vi "niDTS BT INSTR TX Configure ModAcc.vi"(8 "error in (no error)":errorcluster, 11 "niDTS BT INSTR TX in":refnum<class "niDTS BT INSTR TX.lvclass">) -> (0 "error out":errorcluster, 3 "niDTS BT INSTR TX out":refnum<class "niDTS BT INSTR TX.lvclass">)   [LabVIEW 2015, in "niDTS BT.lvlib" / "niDTS BT INSTR TX.lvclass"]
doc: "Sets:\n\n* TriggerThreshold\n* Trigger Source\n* MinQuietTimeDuration\n* TriggerTimeout"
uses:
  niDTS BT INSTR TX.lvclass
  niDTS BT INSTR TX.lvclass/niDTS BT INSTR TX.ctl
  RiviInstDriver/niRfsaBT/Objects/niRfsaBt.lvclass
  RiviInstDriver/InstDriver/Objects/InstDriver.lvclass
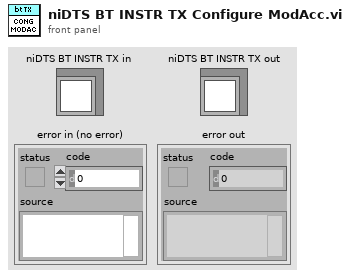
[diagram p1: front panel]
types:
  T1 = typedef "niRfsaBT.lvclass/niRfsaBT INC Handle.ctl" = refnum<data-value>
  T2 = typedef "niDTS BT.lvlib/niDTS BT Tx Test INC Modulation Characteristics.ctl" = enum16{"DF1", "DF2", "BOTH"}
  T3 = enum16{"RMS", "LOG", "SCALAR", "MAX", "MIN", "VECTOR"}
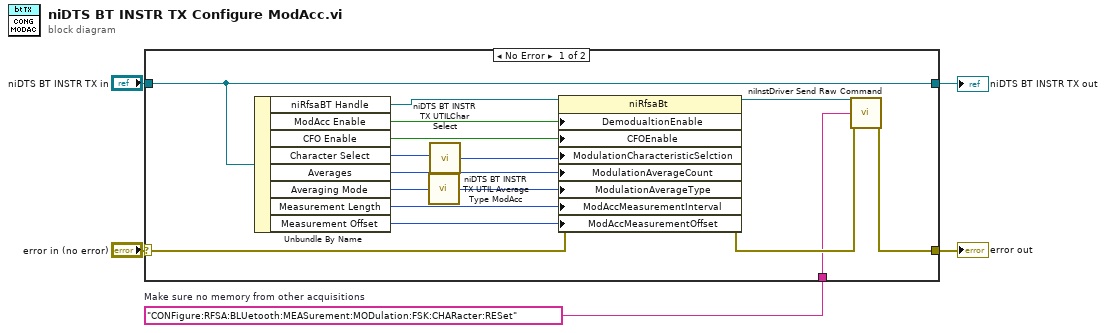
[diagram p0: block diagram]
diagram:
  w1 = "CONFigure:RFSA:BLUetooth:MEASurement:MODulation:FSK:CHARacter:RESet"  # Make sure no memory from other acquisitions
  n1 = case shown="No Error" "error in (no error)" {
    selector: "error in (no error)" -> [w21 w23]
    tunnel: [w7 w23] -> w4
    tunnel: "niDTS BT INSTR TX in" -> [w19 w22]
    tunnel: [w19 w22] -> w2
    tunnel: w1 -> [w6 _]
    frame No Error {
      n2 = Unbundle By Name(w19) -> ("niRfsaBT Handle"=w20:T1, "ModAcc Enable"=w18:bool, "CFO Enable"=w17:bool, "Character Select"=w15:T2, "Averages"=w16:i32, "Averaging Mode"=w14:T3, "Measurement Length"=w13:i32, "Measurement Offset"=w12:i32)
      n3 = call "niDTS BT INSTR TX UTIL Average Type ModAcc.vi"("Average In"=w14) -> ("Average Out"=w10:enum16{"RMS", "MAX", "MIN"})  [unwired: 14 in]
      n4 = call "niDTS BT INSTR TX UTILChar Select.vi"("Character Select"=w15) -> ("ModulationCharacteristicSelction"=w11:enum16{"DF1", "DF2"})  [unwired: 14 in]
      n5 = property class="niRfsaBt"(reference=w20, error in=w21, "DemodualtionEnable"=w18, "CFOEnable"=w17, "ModulationCharacteristicSelction"=w11, "ModulationAverageCount"=w16, "ModulationAverageType"=w10, "ModAccMeasurementInterval"=w13, "ModAccMeasurementOffset"=w12) -> (reference out=w9:T1, error out=w8:errorcluster)
      n6 = call "niInstDriver Send Raw Command.vi"("InstDriver Handle in"=w9, "Command"=w6, "error in (no error)"=w8) -> ("error out"=w7:errorcluster)  [unwired: 11 in, 1 out]
    }
    frame Error {
    }
  }
  "error out" <- w4
  "niDTS BT INSTR TX out" <- w2
